vi "Generate Y.vi"(8 "error in (no error)":errorcluster, 10 "SLAM In":T2) -> (0 "error out":errorcluster, 1 "Reobserved Array":bool[](array[boolean]), 2 "SLAM Out":T2, 3 "Y":T1)   [LabVIEW 2009]
uses:
  Controls/SLAM.ctl
  <vilib>/Analysis/Matrix/Datatypes/RealMatrix.ctl
  <vilib>/Analysis/baseanly.llb/Real A x B.vi
  <vilib>/Analysis/Matrix/NI_Matrix.lvlib
  <vilib>/Analysis/NI_AALBase.lvlib
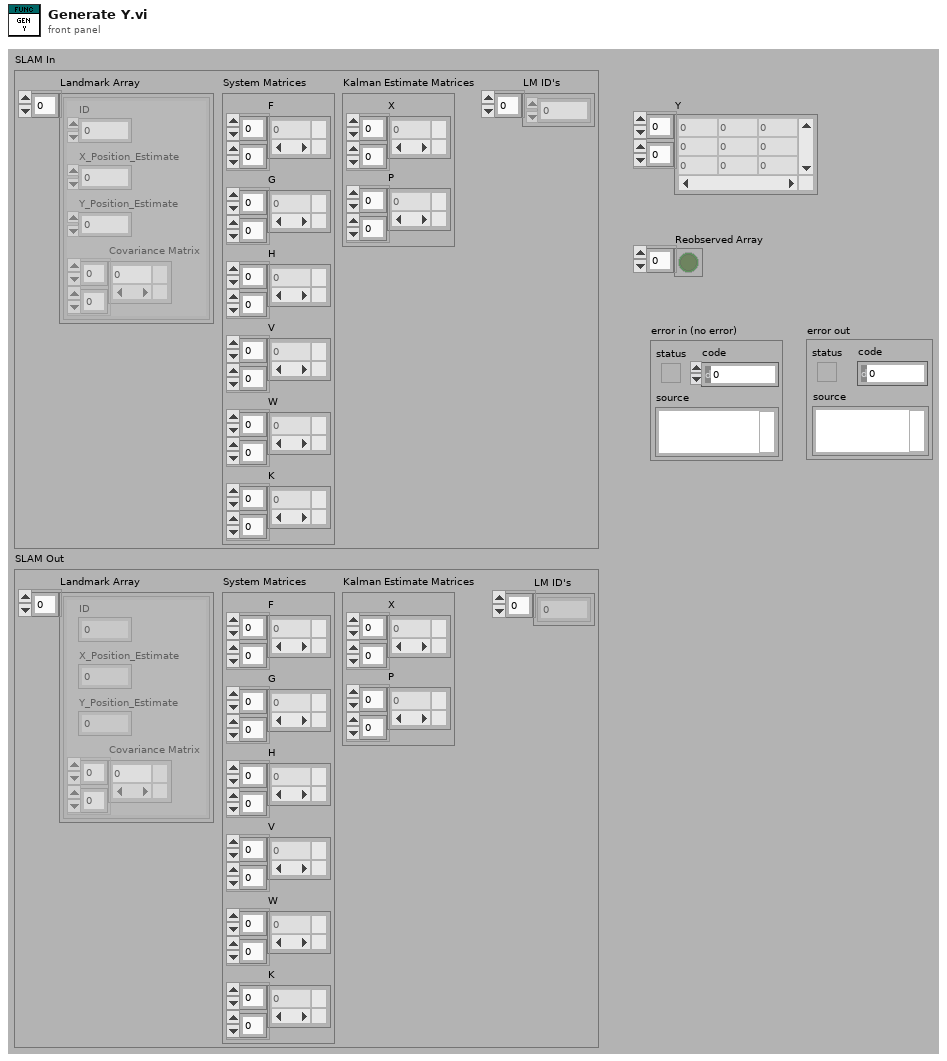
[diagram p1: front panel]
types:
  T1 = typedef "NI_Matrix.lvlib/RealMatrix.ctl" = dbl[][]
  T2 = typedef "SLAM.ctl" = cluster{"Landmark Array":cluster{"ID":dbl, "X_Position_Estimate":dbl, "Y_Position_Estimate":dbl, "Covariance Matrix":T1}[], "System Matrices":cluster{"F":T1, "G":T1, "H":T1, "V":T1, "W":T1, "K":T1}, "Kalman Estimate Matrices":cluster{"X":T1, "P":T1}, "LM ID's":dbl[]}
  T3 = cluster{"ID":dbl, "X_Position_Estimate":dbl, "Y_Position_Estimate":dbl, "Covariance Matrix":T1}[]
  T4 = cluster{"ID":dbl, "X_Position_Estimate":dbl, "Y_Position_Estimate":dbl, "Covariance Matrix":T1}
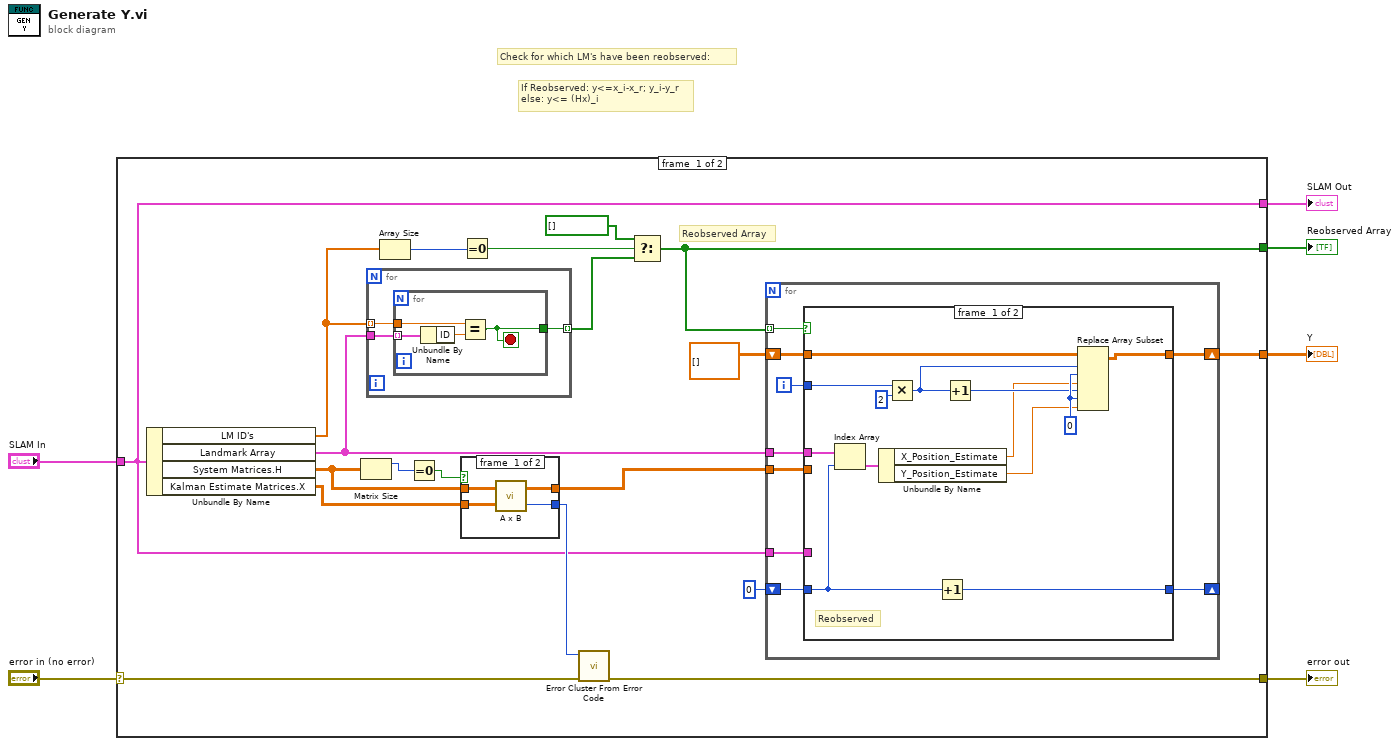
[diagram p0: block diagram]
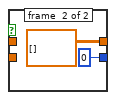
[diagram p2: hidden frame]
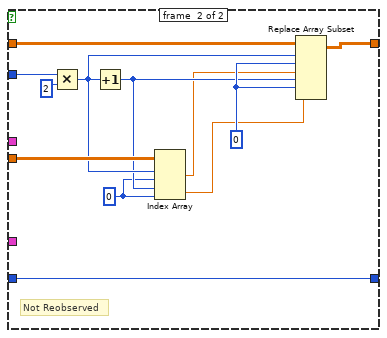
[diagram p3: hidden frame]
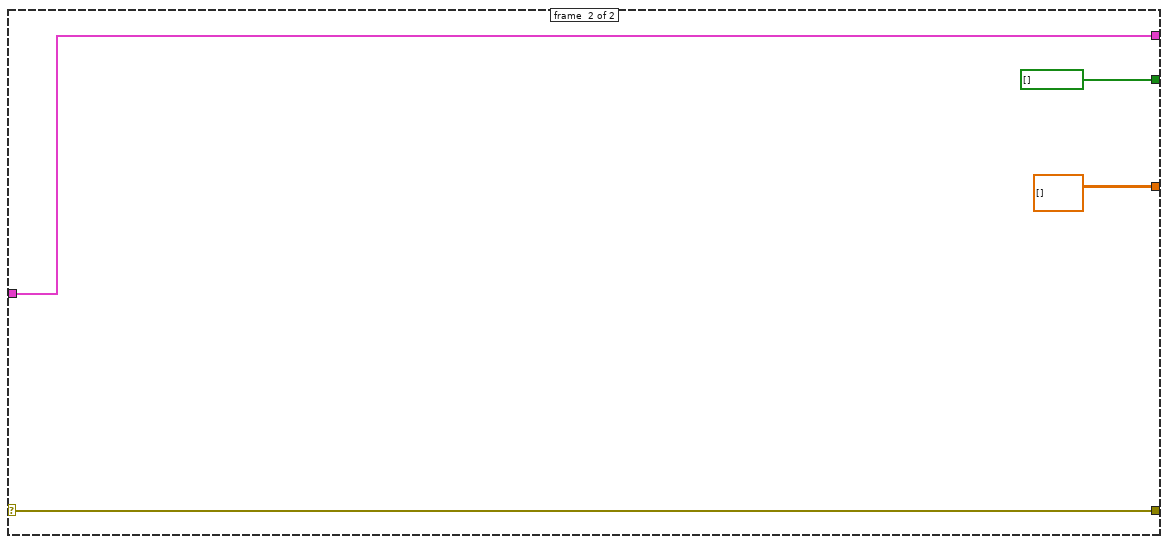
[diagram p4: hidden frame]
diagram:
  # "If Reobserved: y<=x_i-x_r; y_i-y_r\nelse: y<= (Hx)_i"
  # "Check for which LM's have been reobserved:"
  n1 = case shown="No Error" "error in (no error)" {
    selector: "error in (no error)" -> [w19 w75]
    tunnel: [w20 T1 [] ("matrix")] -> w6
    tunnel: [w7 w75] -> w5
    tunnel: "SLAM In" -> [w8 w76]
    tunnel: [w8 w76] -> w2
    tunnel: [w9 bool[] []] -> w1
    frame #0 {
      # "Reobserved Array"
      n2 = Unbundle By Name(w8) -> ("LM ID's"=w14:dbl[], "Landmark Array"=w25:T3, "System Matrices.H"=w17:T1, "Kalman Estimate Matrices.X"=w23:T1)
      n3 = Matrix Size(0:w17) -> (1:w16:i32)  [unwired: 1 out]
      n4 = for {
        tunnel: w25 -> [w68]
        tunnel: w14 -> [w67] mode=indexing
        tunnel: [w66] -> w11 mode=indexing
        n5 = for {
          tunnel: w68 -> [w72] mode=indexing
          tunnel: w67 -> [w70]
          tunnel: [w69] -> w66
          stop <- w69 stop-if-true
          n6 = Unbundle By Name(w72) -> ("ID"=w71:dbl)
          n7 = Equal?(x=w70, y=w71) -> (x = y?=w69:bool)
        }
      }
      n8 = Array Size(array=w14) -> (size(s)=w13:i32)
      n9 = Equal To 0?(x=w16) -> (x = 0?=w15:bool)
      n10 = case shown="False" w15 {
        tunnel: w17 -> [w29 _]
        tunnel: w23 -> [w28 _]
        tunnel: [w27 0 ("error")] -> w22
        tunnel: [w26 T1 [] ("A x B")] -> w21
        frame #0 {
          n11 = call-poly <vilib>:"A x B.vi"("B"=w28, "A"=w29) -> ("error"=w27:i32, "A x B"=w26:T1)
        }
        frame #1 {
        }
      }
      n12 = Equal To 0?(x=w13) -> (x = 0?=w12:bool)
      n13 = call <vilib>:"Error Cluster From Error Code.vi"("error in (no error)"=w19, "error code (0)"=w22) -> ("error out"=w7:errorcluster)  [unwired: 7 in]
      n14 = Select(t=bool[] [], s=w12, f=w11) -> (s? t:f=w9:bool[])
      n15 = for {
        tunnel: w9 -> [w40] mode=indexing
        tunnel: w25 -> [w39]
        shift-right: [w36] -> w20
        shift-left: T1 [] ("matrix") -> [w37]
        tunnel: w21 -> [w35]
        shift-right: [w33] -> _
        shift-left: 0 ("index") -> [w34]
        tunnel: w8 -> [w32]
        i -> [w38]
        n16 = case shown="True" w40 {
          tunnel: w39 -> [w53 _]
          tunnel: w38 -> [w48 w62]
          tunnel: w37 -> [w51 w65]
          tunnel: [w50 w64] -> w36
          tunnel: w35 -> [_ w60]
          tunnel: w34 -> [w44 w54]
          tunnel: [w43 w54] -> w33
          tunnel: w32 -> [_ _]
          frame #0 {
            w49 = 0 ("index (col)")
            # "Reobserved"
            n17 = Index Array(array=w53, index=w44) -> (element=w52:T4)
            n18 = Unbundle By Name(w52) -> ("X_Position_Estimate"=w42:dbl, "Y_Position_Estimate"=w41:dbl)
            n19 = Multiply(x=w48, y=2) -> (x*y=w46:i32)
            n20 = Increment(x=w44) -> (x+1=w43:i32)
            n21 = Increment(x=w46) -> (x+1=w45:i32)
            n22 = Replace Array Subset(array=w51, new element #1=w42, index (row) #1=w46, index (col) #1=w49, new element #2=w41, index (row) #2=w45, index (col) #2=w49) -> (w50:T1)
          }
          frame #1 {
            w57 = 0 ("column 1")
            w63 = 0 ("index (col)")
            # "Not Reobserved"
            n23 = Multiply(x=w62, y=2) -> (x*y=w59:i32)
            n24 = Increment(x=w59) -> (x+1=w58:i32)
            n25 = Index Array(array=w60, index (row) #1=w59, index (col) #1=w57, index (row) #2=w58, index (col) #2=w57) -> (element #1=w56:dbl, element #2=w55:dbl)
            n26 = Replace Array Subset(array=w65, new element #1=w56, index (row) #1=w59, index (col) #1=w63, new element #2=w55, index (row) #2=w58, index (col) #2=w63) -> (w64:T1)
          }
        }
      }
    }
    frame #1 {
    }
  }
  "SLAM Out" <- w2
  "Y" <- w6
  "error out" <- w5
  "Reobserved Array" <- w1
